vi "FPGA-7842R-Control V2.vi"(0 "Waveform Data":T4, 1 "Current Frame":u16, 2 "Action":T5=enum."Exit", 3 "Laser On Time (Ticks)":u8=13, 5 "Laser Controls":T1 {"STED Power (V)" scale=0.0..10.0}, 7 "Manual Controls":T3={"Galvo 1 Position (I16)"=-280, "Galvo 2 Position (I16)"=-280, "X Axis Voltage (I16)"=0, "Y Axis Voltage (I16)"=0, "Z Axis Voltage (I16)"=0, "Res Mirror Amp (I16)"=0, "Res Mirror Mute"=FALSE, "Upper Shutter"=FALSE, "Lower Shutter"=FALSE}, 9 "Image Acquisition Parameters":T2={"Scan Type"=enum."Sample Scanning", "Scan Mode"=enum."XY", "Fast Axis Frequency (Hz)"=100.0, "Image Format"=128, "Line Accumulations"=1, "Frames Per Capture"=1, "Frames Accumulations"=1, "Image Dimension (um)"=[], "Number of Z Steps"=1, "Z Steps Size (um)"=1.0, "Pixel Size (nm)"=[], "Customized Image Format"=[]} {"Z Steps Size (um)" min=0.0; "Number of Z Steps" min=1; "Frames Accumulations" min=1; "Frames Per Capture" min=1; "Line Accumulations" min=1; "Image Format" items=["64 x 64"=64, "128 x 128"=128, "256 x 256"=256, "512 x 512"=512, "1024 x 1024"=1024, "2048 x 2048"=2048, "Customized..."=0]}, 11 "Initialize":bool, 12 "Unused Axis Offset (I16)":i16, 14 "Laser Delay (Ticks)":u8=6) -> (4 "Shutter Status":cluster{"US Status":bool, "LS Status":bool}, 15 "Initalized":bool)   [LabVIEW 2014]
uses:
  FPGA-7842R-Reference.ctl
  Waveform Data.ctl
  Manual Controls V2.ctl
  Type Defs/Image Acquisition Parameters.ctl
  Laser Controls.ctl
  <vilib>/FPGAPlugInAG/PCIe-7841R/niLvFpga_Open_PCIe-7841R.vi
  <vilib>/Utility/error.llb/Error Cluster From Error Code.vi
  <vilib>/rvi/errors/niLvFpgaAdjustHostInterfaceError.vi
  <vilib>/FPGAPlugInAG/PCIe-7841R/niLvFpga_Run_PCIe-7841R.vi
  <vilib>/FPGAPlugInAG/PCIe-7841R/niLvFpga_Close_PCIe-7841R.vi
  <vilib>/rvi/interface/nirviOpenFPGA/nirviOpenFPGA.xnode
  FPGA Bitfiles/MainSTEDFPGAProj_FPGATarget_WaveformandLaser_sIm2Xng7ncM.lvbitx
  FPGA Target VIs/FPGA-7841R/Waveform and Laser Controls V7.vi
  <vilib>/rvi/interface/nirviReadWriteControl/nirviReadWriteControl.xnode
  FPGA Target VIs/FPGA-7841R/Waveform Scan Parameters.ctl
  <vilib>/rvi/interface/nirviMethod/nirviMethod.xnode
  <vilib>/rvi/interface/nirviCloseFPGA/nirviCloseFPGA.xnode
  NiFpgaLv.dll
panel:
  # "Length"
  # "Height"
  # "XY"
  # "Z"
  # "Length"
  # "Height"
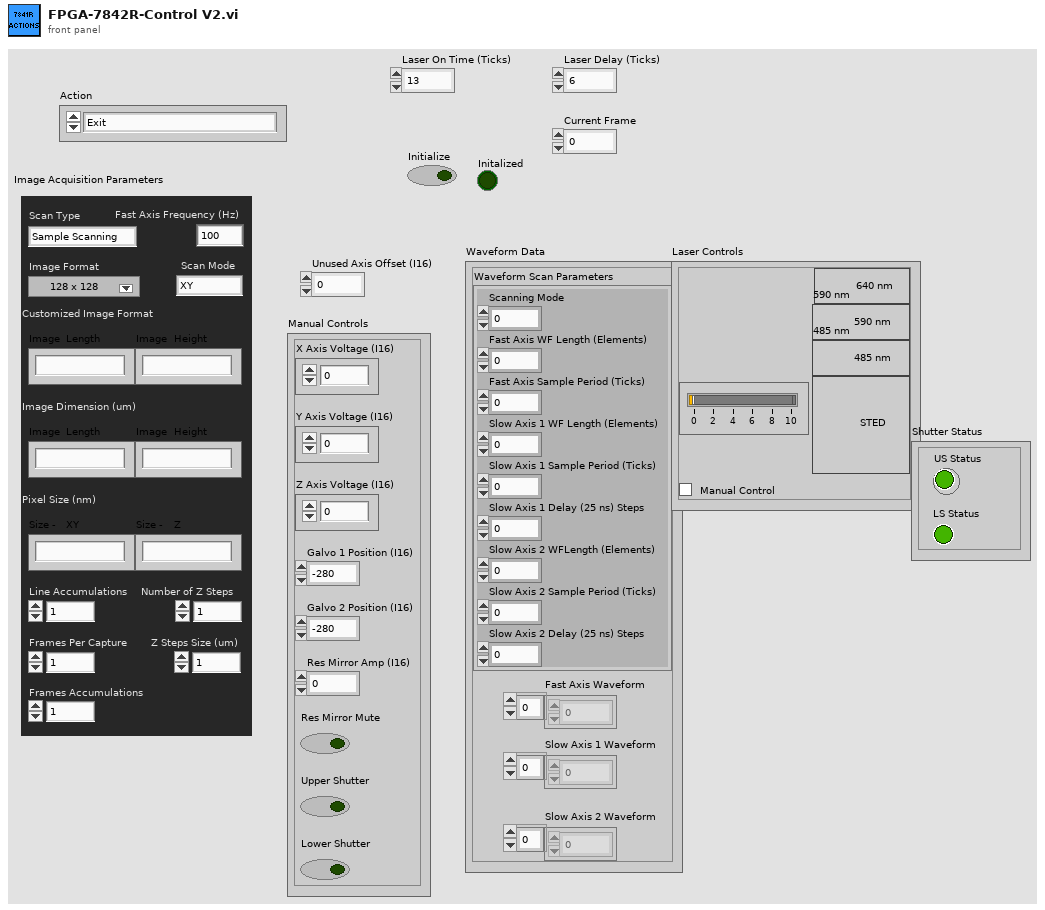
[diagram p1: front panel]
types:
  T1 = typedef "Laser Controls.ctl" = cluster{"STED Power (V)":dbl, "STED":bool, "650 nm":bool, "590 nm":bool, "485 nm":bool, "Manual Control":bool}
  T2 = typedef "Image Acquisition Parameters.ctl" = cluster{"Scan Type":enum16{"Sample Scanning", "Beam Scanning"}, "Scan Mode":enum16{"XY", "XZ", "YZ", "XYZ"}, "Fast Axis Frequency (Hz)":dbl, "Image Format":u16, "Line Accumulations":u16, "Frames Per Capture":u16, "Frames Accumulations":u16, "Image Dimension (um)":dbl[], "Number of Z Steps":u16, "Z Steps Size (um)":dbl, "Pixel Size (nm)":dbl[], "Customized Image Format":dbl[]}
  T3 = typedef "Manual Controls V2.ctl" = cluster{"Galvo 1 Position (I16)":i16, "Galvo 2 Position (I16)":i16, "X Axis Voltage (I16)":i16, "Y Axis Voltage (I16)":i16, "Z Axis Voltage (I16)":i16, "Res Mirror Amp (I16)":i16, "Res Mirror Mute":bool, "Upper Shutter":bool, "Lower Shutter":bool}
  T4 = typedef "Waveform Data.ctl" = cluster{"Waveform Scan Parameters":cluster{"Scanning Mode":u8, "Fast Axis WF Length (Elements)":i32, "Fast Axis Sample Period (Ticks)":u32, "Slow Axis 1 WF Length (Elements)":i32, "Slow Axis 1 Sample Period (Ticks)":u32, "Slow Axis 1 Delay (25 ns) Steps":i32, "Slow Axis 2 WFLength (Elements)":i32, "Slow Axis 2 Sample Period (Ticks)":u32, "Slow Axis 2 Delay (25 ns) Steps":i32}, "Fast Axis Waveform":dbl[], "Slow Axis 1 Waveform":dbl[], "Slow Axis 2 Waveform":dbl[]}
  T5 = typedef "FPGA-7842R-Reference.ctl" = enum16{"Stage Control", "Laser Control", "Unused Axis I16", "Exit", "Set Res Mirror", "Set Galvo", "Current Frame for Capture", "Default", "Close FPGA", "Stop Waveforms", "Start Waveforms", "Shutter Control", "Initialize"}
  T6 = cluster{"Scanning Mode":u8, "Fast Axis WF Length (Elements)":i32, "Fast Axis Sample Period (Ticks)":u32, "Slow Axis 1 WF Length (Elements)":i32, "Slow Axis 1 Sample Period (Ticks)":u32, "Slow Axis 1 Delay (25 ns) Steps":i32, "Slow Axis 2 WFLength (Elements)":i32, "Slow Axis 2 Sample Period (Ticks)":u32, "Slow Axis 2 Delay (25 ns) Steps":i32}
  T7 = cluster{"Res Mirror Amp (I16)":i16, "Res Mirror Mute":bool}
  T8 = typedef "Scan Parameters.ctl" = cluster{"Fast_Ax_Amp_V":dbl, "Fast_Ax_Off_V":dbl, "Slow_Ax_Amp_V":dbl, "Slow_Ax_Off_V ":dbl, "Slow_Ax_Max_V_VperS":dbl, "Slow_Ax1_Del25ns":i32, "Slow_Ax2_Del25ns":i32, "Stage_X_Off_V":dbl, "Stage_Y_Off_V":dbl, "Stage_Z_Off_V":dbl, "Galvo1_Off_V":dbl, "Galvo2_Off_V":dbl, "Last_Scan_Mode":enum16{"XY", "XZ", "YZ", "XYZ"}, "Current_Scan_Mode":enum16{"XY", "XZ", "YZ", "XYZ"}, "Fly_Back_Lines":u16, "Linear_Ramp_End":u32, "Z_Step_I16":i16, "Z_Start_I16":i16, "Laser_States _U32":u32, "590_Voltage_I16":i16, "775_AOM_Volt_I16":i16, "Blanking OFF":bool, "Unused_Axis_I16":i16}
  T9 = cluster{"Upper Shutter Status":bool, "Lower Shutter Status":bool}
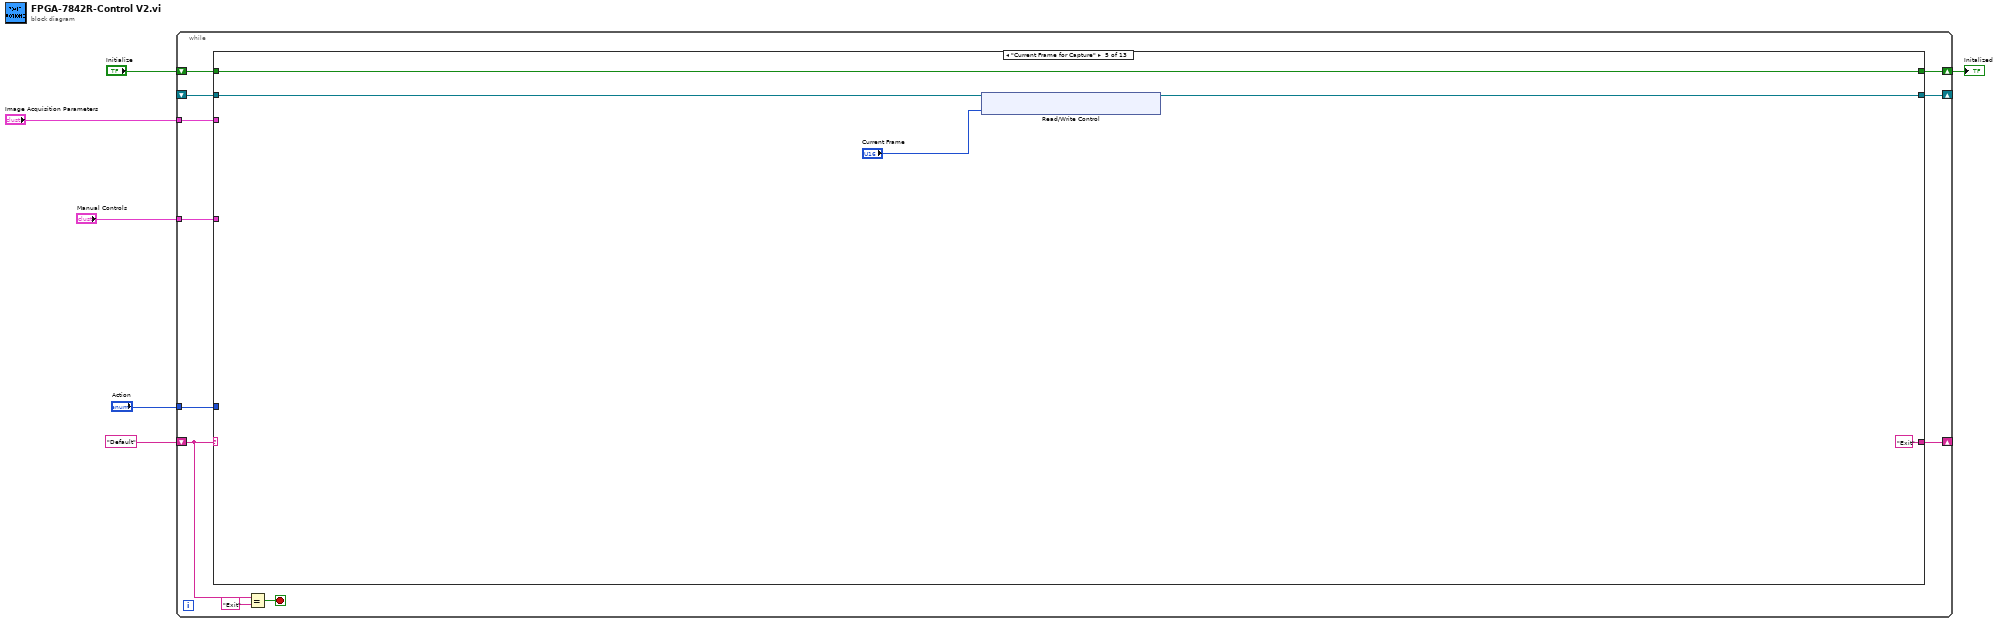
[diagram p0: block diagram]
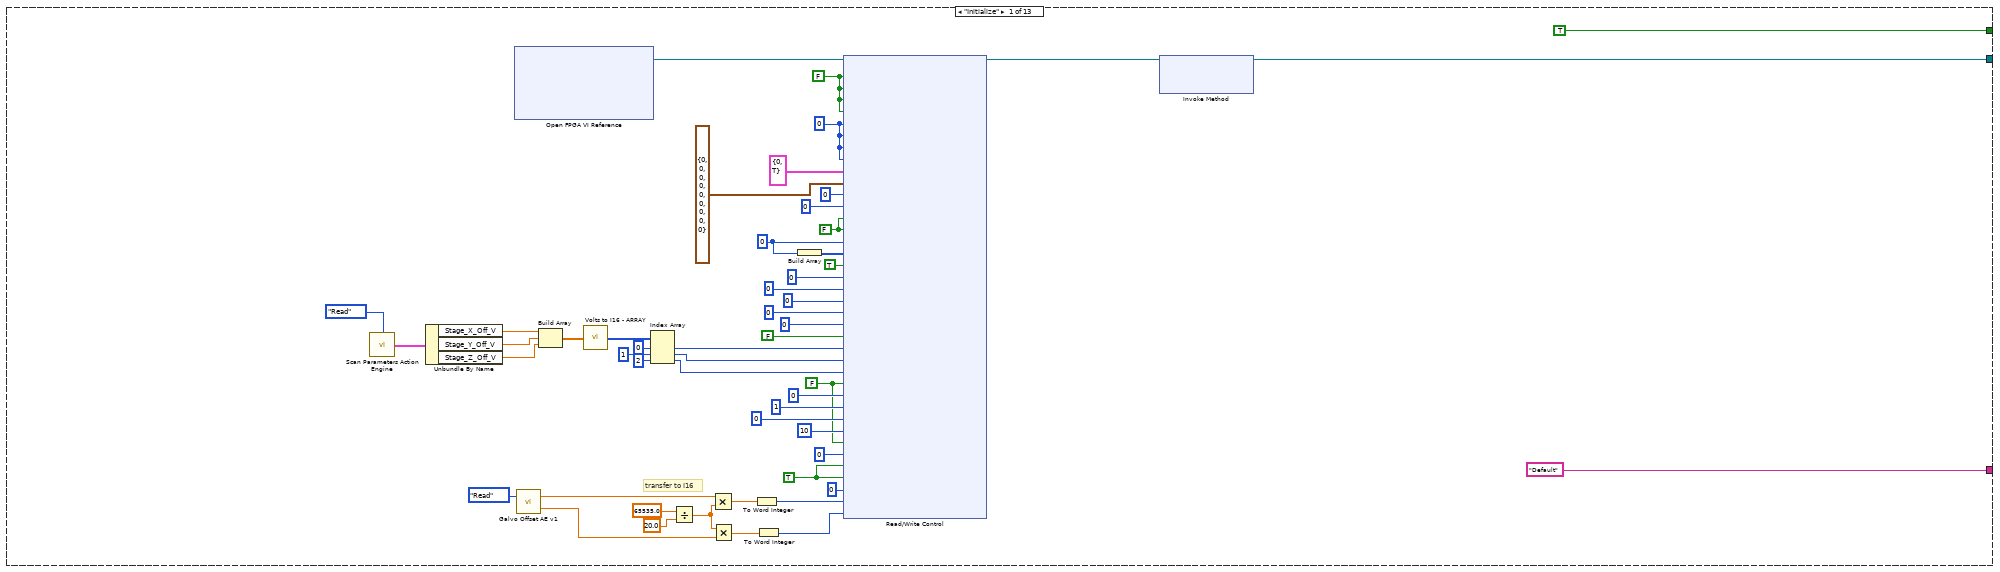
[diagram p2: hidden frame]
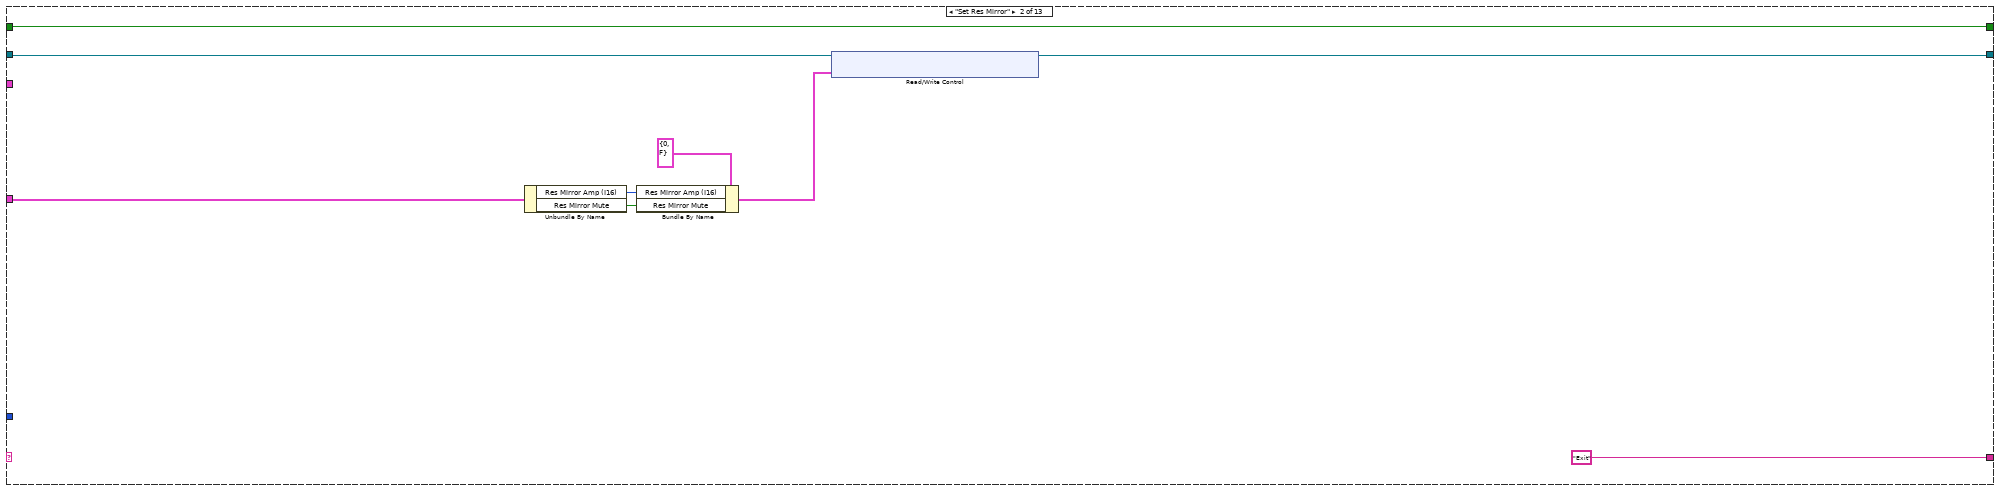
[diagram p3: hidden frame]
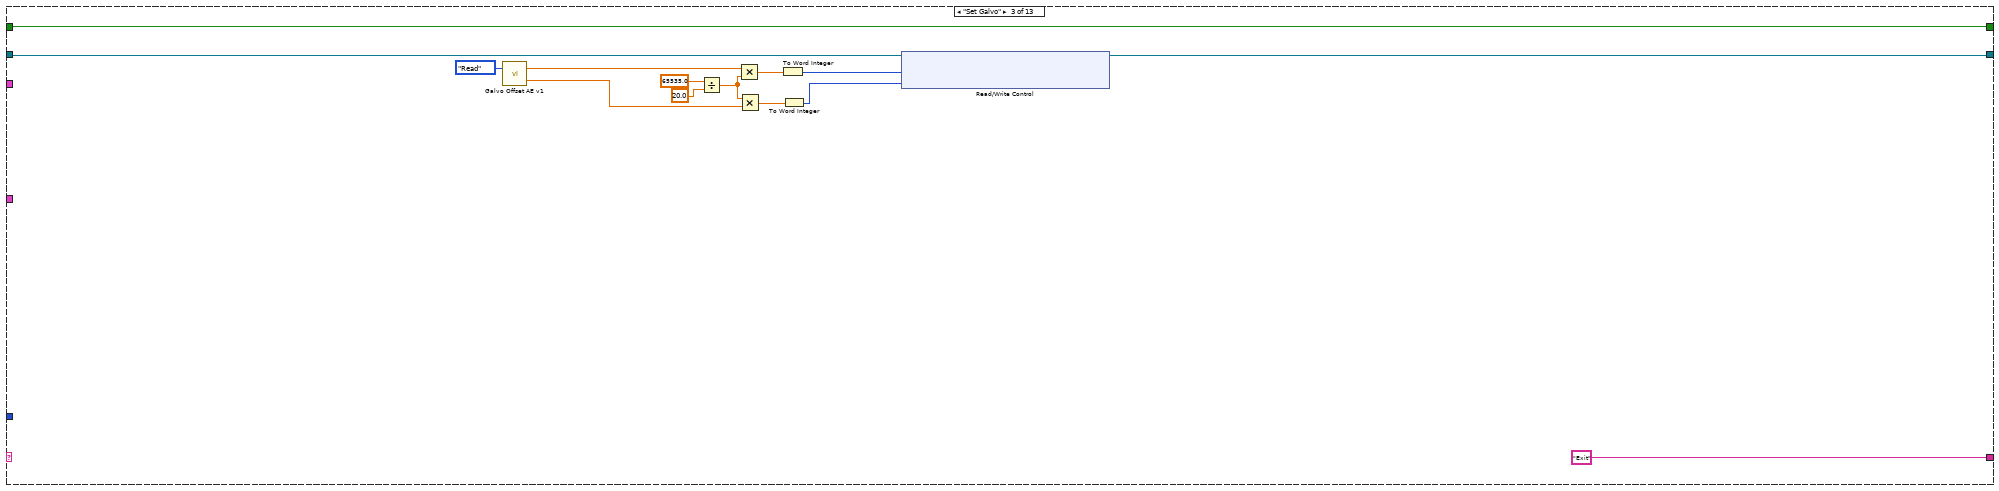
[diagram p4: hidden frame]
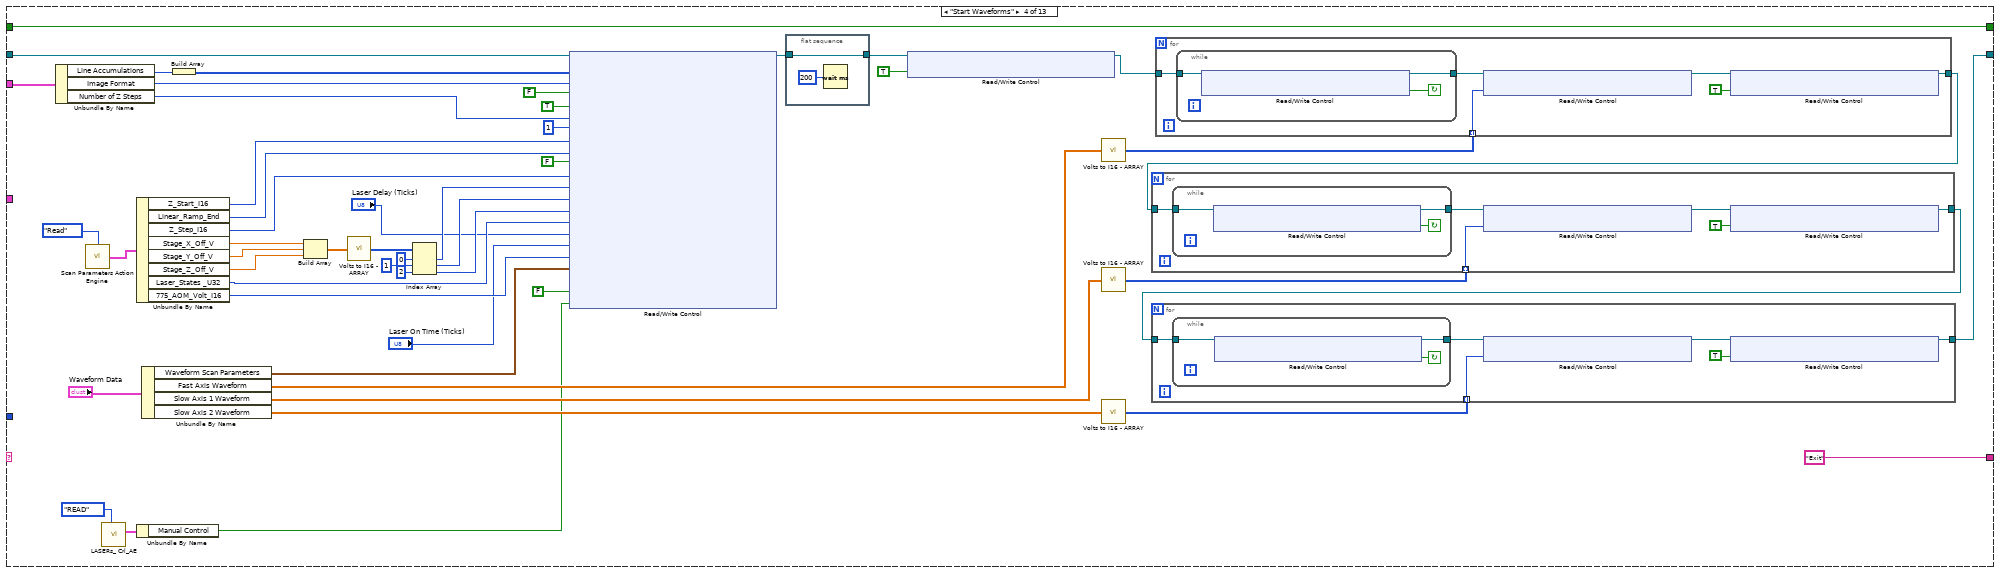
[diagram p5: hidden frame]
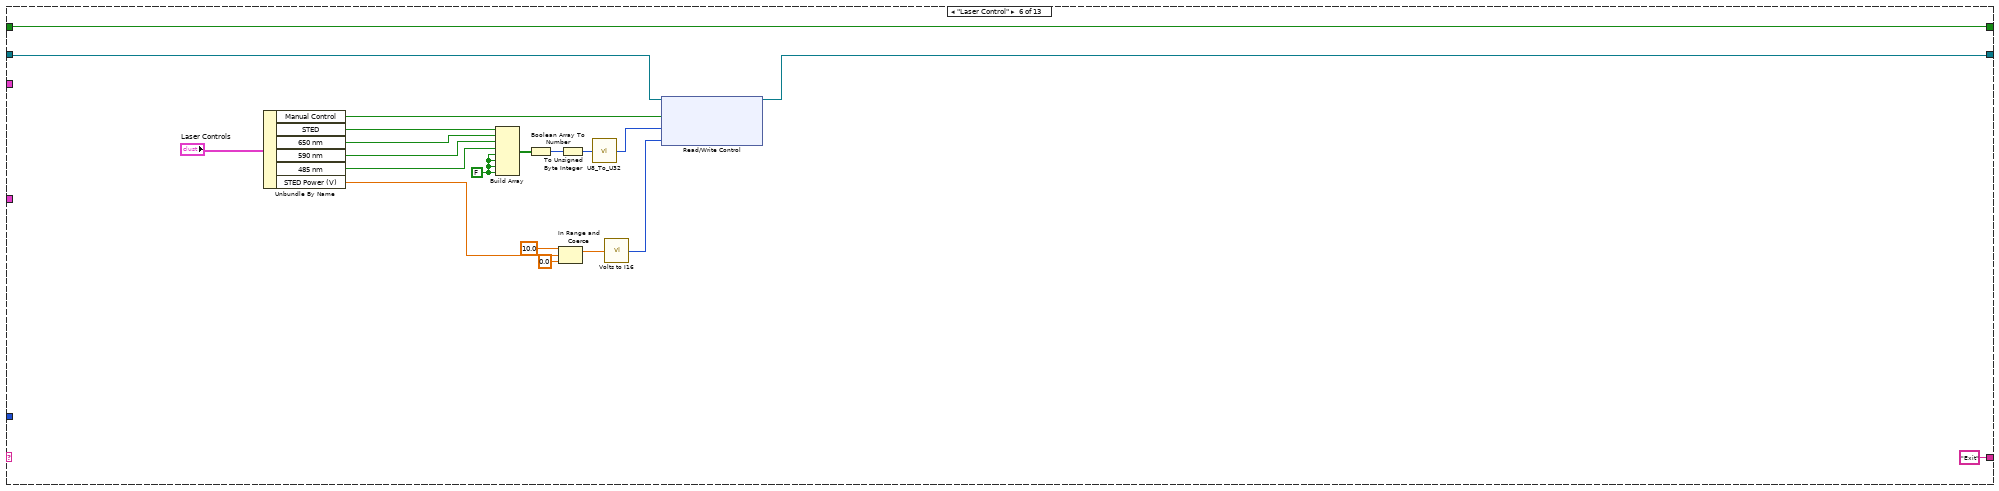
[diagram p6: hidden frame]
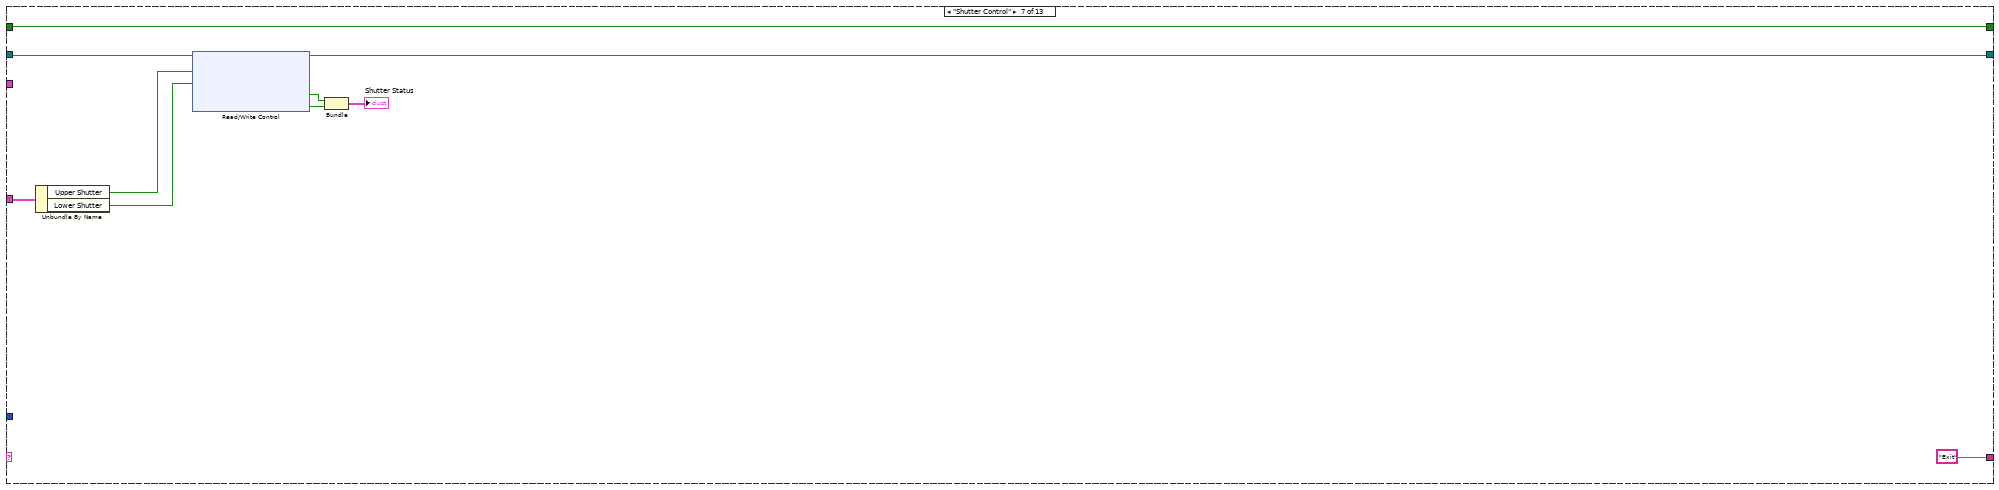
[diagram p7: hidden frame]
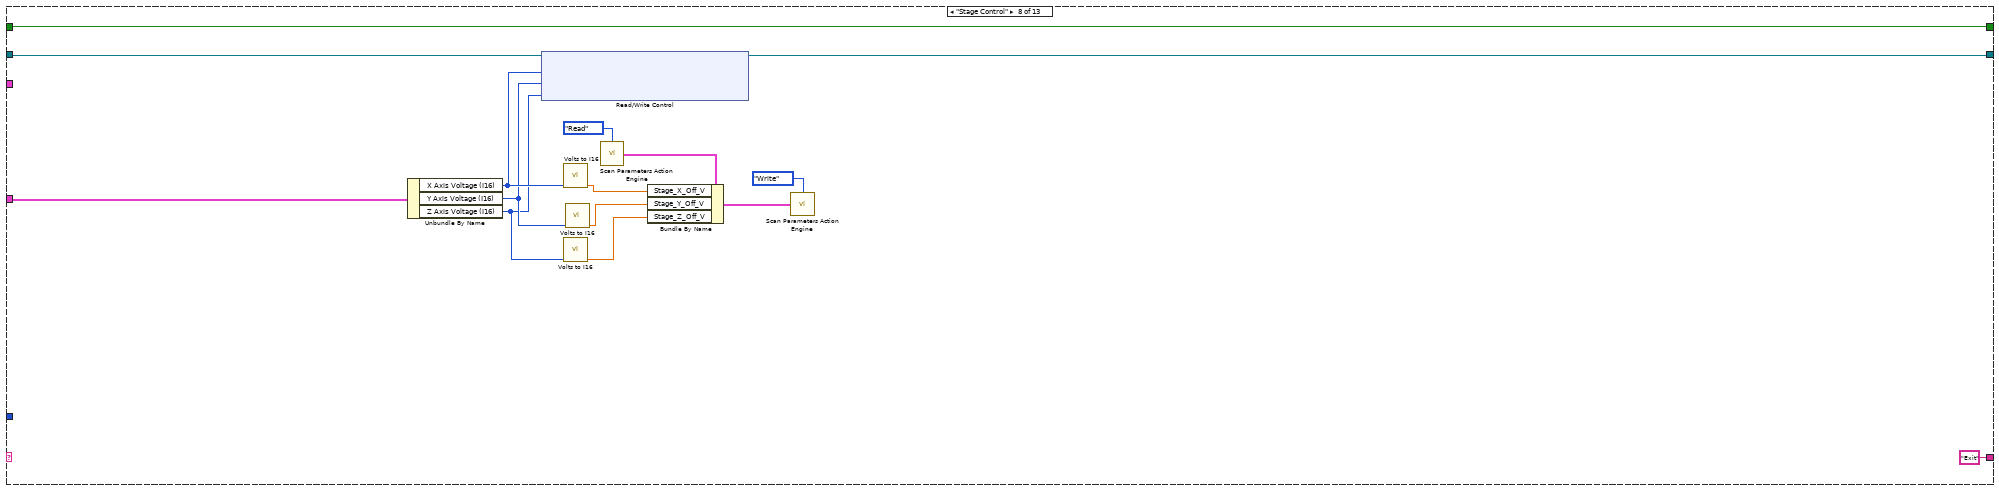
[diagram p8: hidden frame]
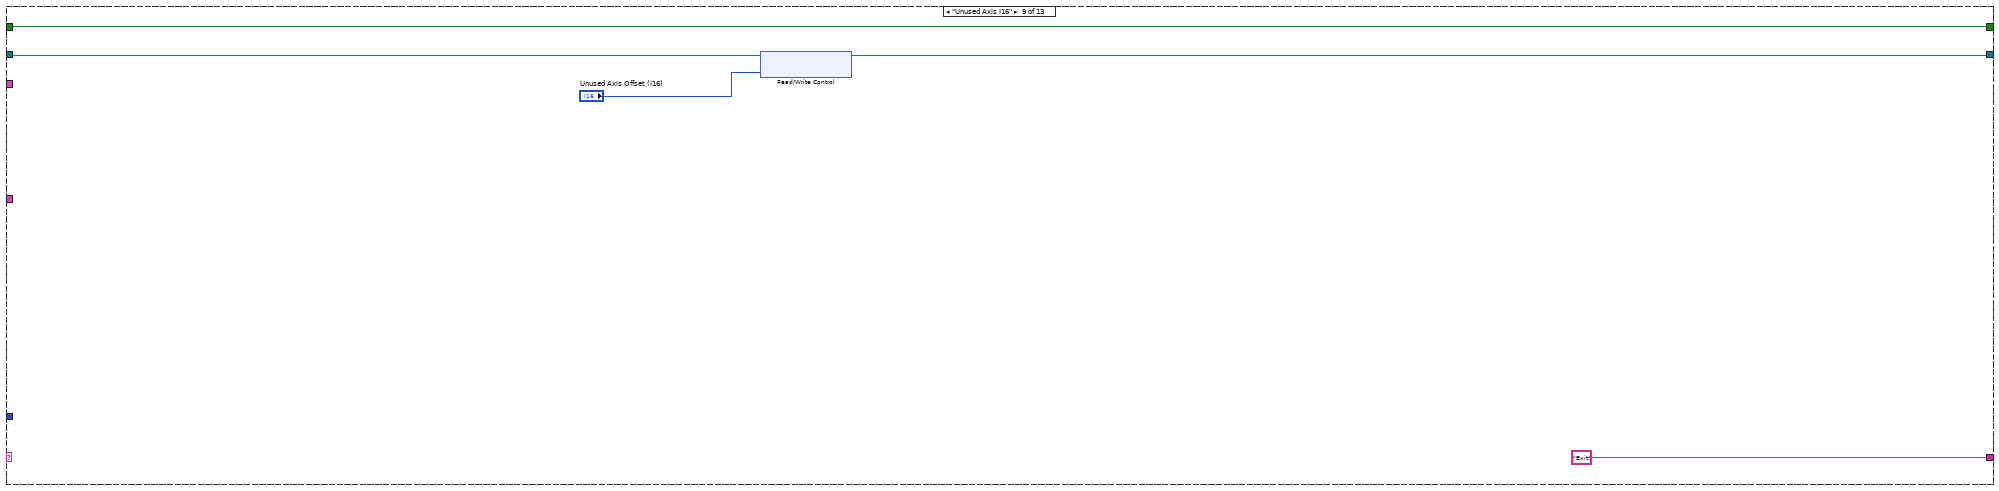
[diagram p9: hidden frame]
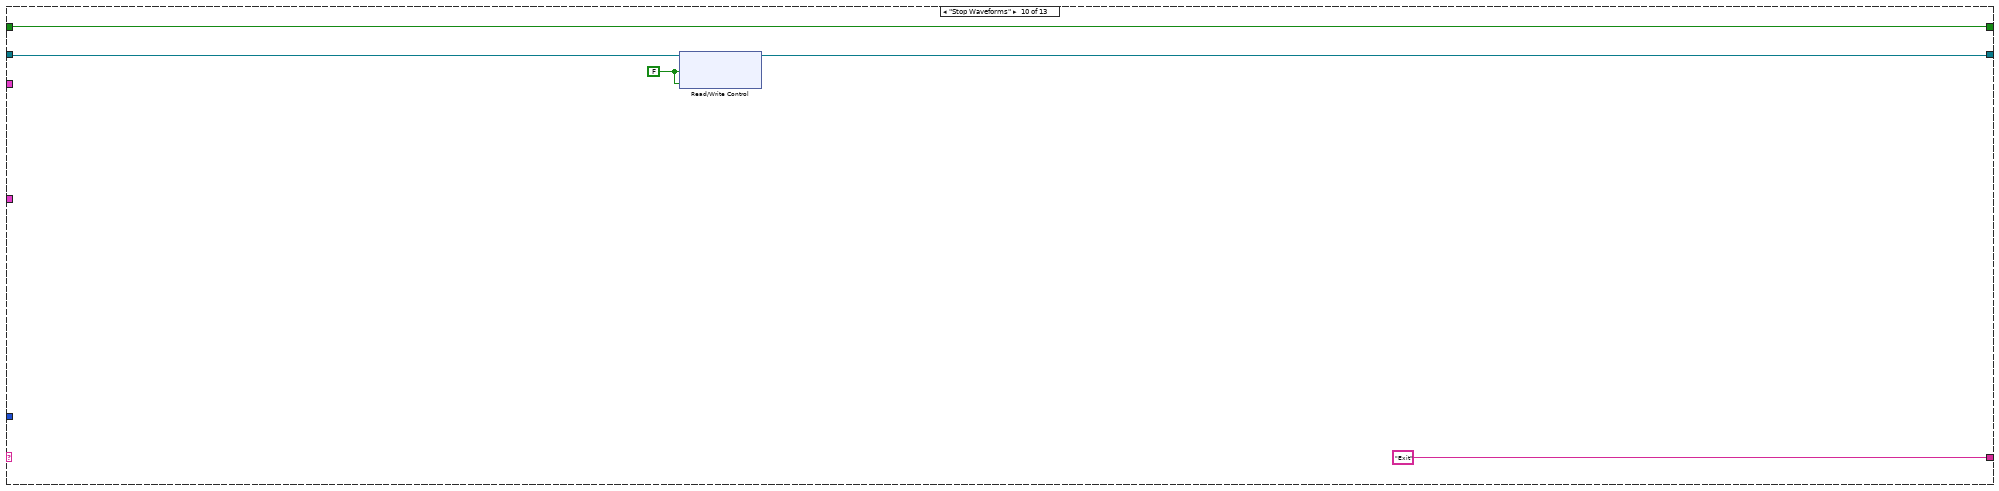
[diagram p10: hidden frame]
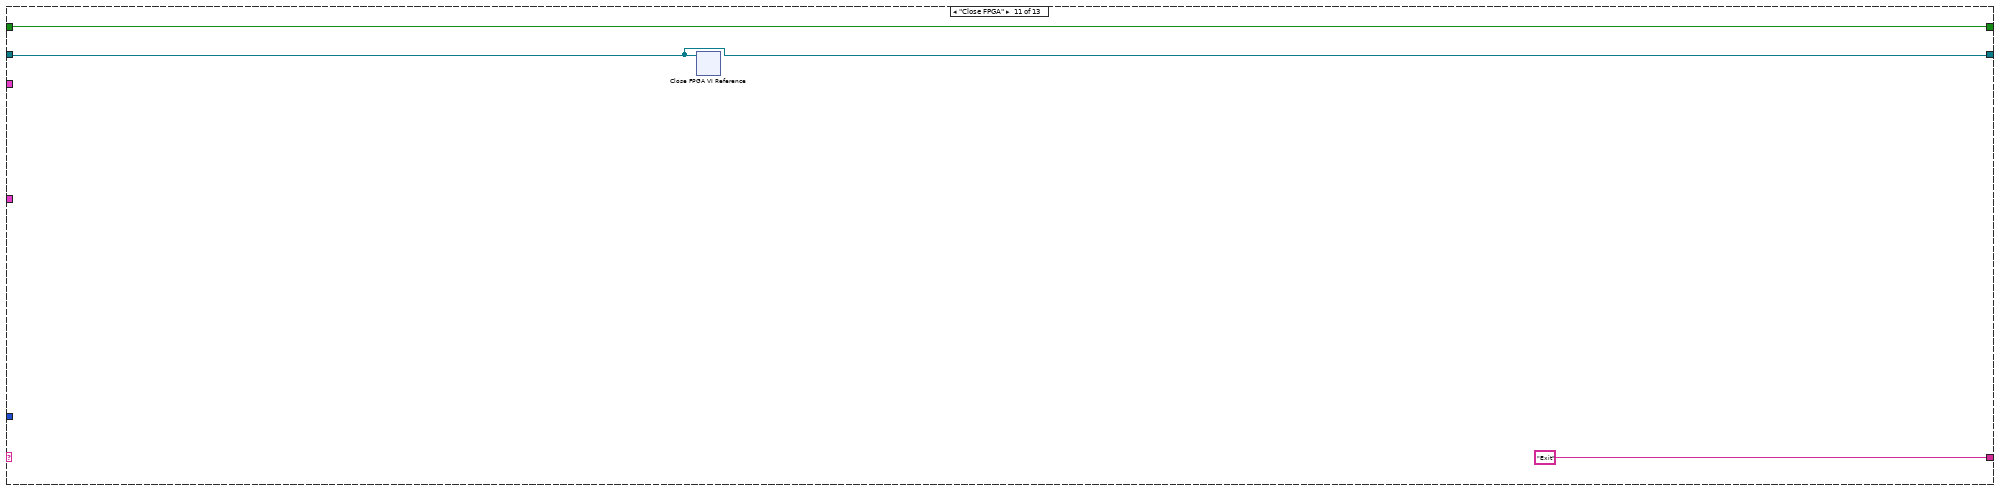
[diagram p11: hidden frame]
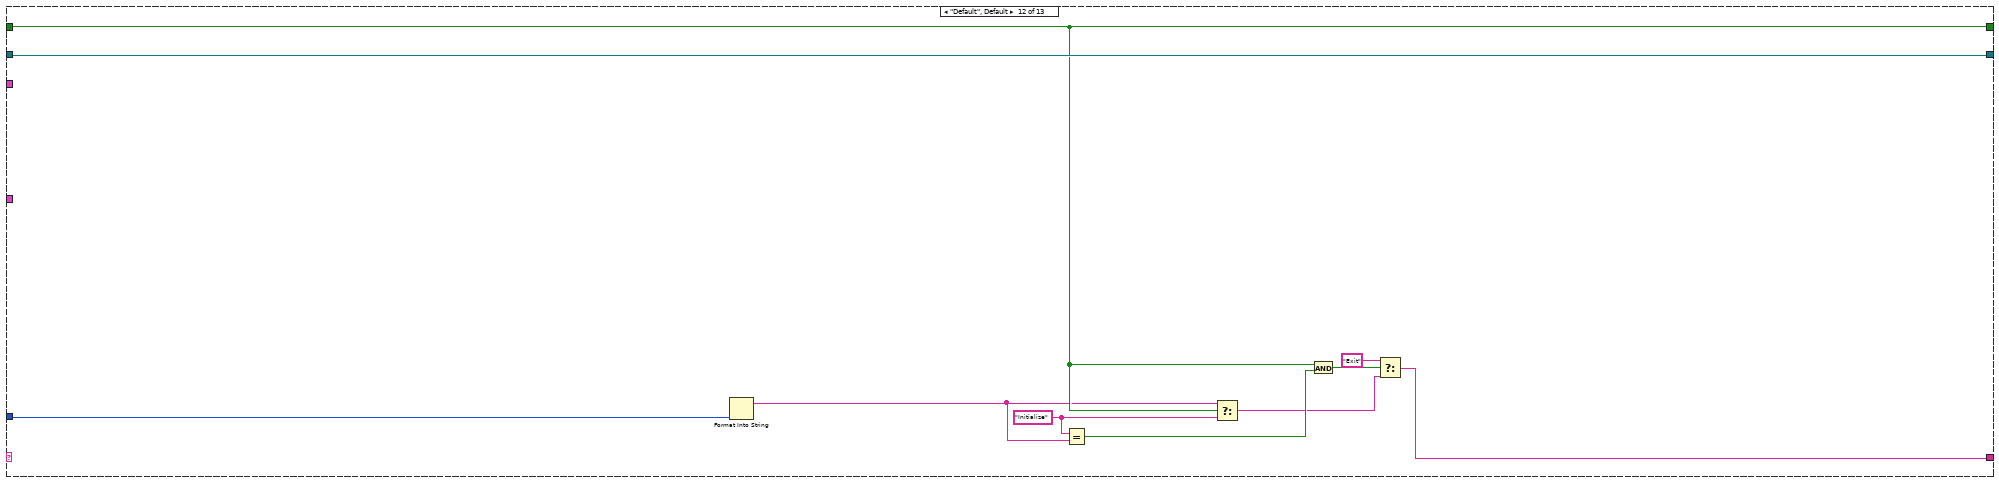
[diagram p12: hidden frame]
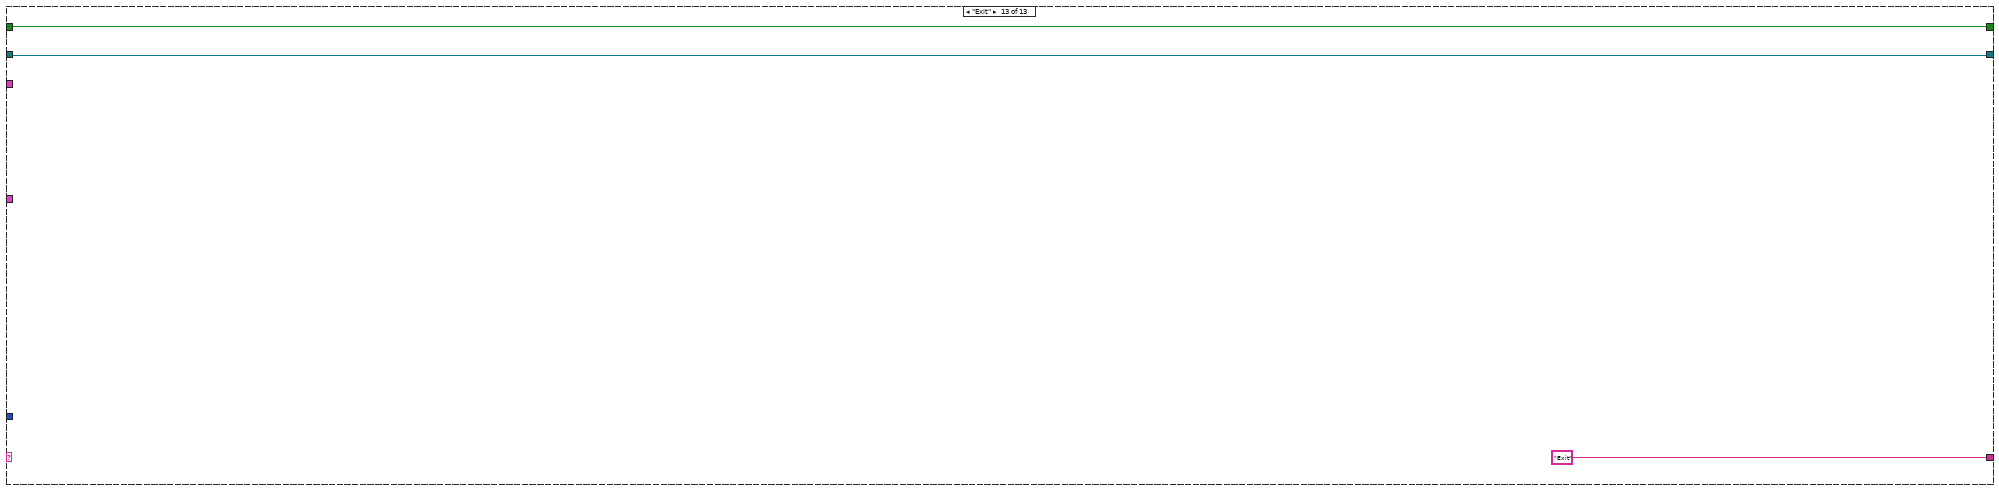
[diagram p13: hidden frame]
diagram:
  n1 = while {
    shift-right: [w17] -> _
    shift-left: _ -> [w16]
    shift-right: [w14] -> _
    shift-left: "Default" -> [w13]
    tunnel: "Action" -> [w15]
    shift-right: [w10] -> w3
    shift-left: "Initialize" -> [w9]
    tunnel: "Manual Controls" -> [w8]
    tunnel: "Image Acquisition Parameters" -> [w7]
    stop <- w11 stop-if-true
    n2 = case shown="\"Current Frame for Capture\"" w13 {
      tunnel: [w60 w75 w89 w132 w175 w193 w205 w218 w224 w231 w233 w245 w247] -> w17
      tunnel: w16 -> [_ w76 w90 w135 w176 w194 w206 w219 w225 w232 w233 w245 w247]
      tunnel: w15 -> [_ _ _ _ _ _ _ _ _ _ _ w244 _]
      tunnel: ["Default" ("f") "Exit" ("f") "Exit" ("f") "Exit" ("f") "Exit" ("f") "Exit" ("f") "Exit" ("f") "Exit" ("f") "Exit" ("f") "Exit" ("f") "Exit" ("f") w238 "Exit" ("f")] -> w14
      tunnel: [TRUE w78 w92 w137 w177 w196 w207 w221 w227 w230 w235 w243 w248] -> w10
      tunnel: w9 -> [_ w78 w92 w137 w177 w196 w207 w221 w227 w230 w235 w243 w248]
      tunnel: w8 -> [_ w74 _ _ _ _ w200 w220 _ _ _ _ _]
      tunnel: w7 -> [_ _ _ w126 _ _ _ _ _ _ _ _ _]
      frame "Initialize" {
        w29 = TRUE ("Upper Shutter Command")
        w31 = FALSE ("Blanking Off/Manual")
        w56 = u16 0 ("Number of Lines")
        w58 = FALSE ("Reset Position Error")
        w69 = i16 0 ("Fast Axis Waveform Element")
        w68 = FALSE ("WF 1 Data Loaded")
        # "transfer to I16"
        n3 = call "Scan Parameters Action Engine.vi"("Action"=enum16{"Read", "Write"}."Read") -> ("Scan Parameters OUT"=w47:T8)  [unwired: 14 in]
        n4 = Unbundle By Name(w47) -> ("Stage_X_Off_V"=w46:dbl, "Stage_Y_Off_V"=w44:dbl, "Stage_Z_Off_V"=w45:dbl)
        n5 = xnode "Open FPGA VI Reference"() -> ("FPGA VI Reference Out"=w59:refnum<k20>)  [unwired: 2 in, 1 out]
        n6 = call "Galvo Offset AE v1.vi"("Action"=enum16{"Read", "Write"}."Read") -> ("Galvo 2 Offset Out"=w18:dbl, "Galvo 1 Offset Out"=w19:dbl)  [unwired: 1 in]
        n7 = Build Array(w46, w44, w45) -> (w43:dbl[])
        n8 = call "Volts to I16 - ARRAY.vi"("Voltage (V)"=w43) -> ("I16"=w42:i16[])  [unwired: 14 in]
        n9 = Index Array(array=w42, index #1=0 ("index"), index #2=1 ("index"), index #3=2 ("index")) -> (element #1=w38:i16, element #2=w36:i16, element #3=w37:i16)
        n10 = Divide(x=65535.0, y=20.0 ("x")) -> (x/y=w23:dbl)
        n11 = Multiply(x=w19, y=w23) -> (x*y=w25:dbl)
        n12 = Multiply(x=w23, y=w18) -> (x*y=w22:dbl)
        n13 = To Word Integer(number=w25) -> (16bit integer=w24:i16)
        n14 = To Word Integer(number=w22) -> (16bit integer=w21:i16)
        n15 = Build Array(w56) -> (w55:u16[])
        n16 = xnode "Read/Write Control"("FPGA VI Reference In"=w59, "WF 1 Data Loaded"=w68, "WF 2 Data Loaded"=w68, "WF 3 Data Loaded"=w68, "Start Waveforms"=w68, "Fast Axis Waveform Element"=w69, "Slow Axis 1 Waveform Element"=w69, "Slow Axis 2 Waveform Element"=w69, "Unused Axis Offset"=w69, "Resonant Mirror"=T7 {"Res Mirror Amp (I16)"=0, "Res Mirror Mute"=TRUE} ("Resoance Mirror"), "Waveform Scan Parameters"=T6 {"Scanning Mode"=0, "Fast Axis WF Length (Elements)"=0, "Fast Axis Sample Period (Ticks)"=0, "Slow Axis 1 WF Length (Elements)"=0, "Slow Axis 1 Sample Period (Ticks)"=0, "Slow Axis 1 Delay (25 ns) Steps"=0, "Slow Axis 2 WFLength (Elements)"=0, "Slow Axis 2 Sample Period (Ticks)"=0, "Slow Axis 2 Delay (25 ns) Steps"=0}, "Galvo 2 Position (I16)"=i16 0, "Galvo 1 Position (I16)"=i16 0, "Reset Position Error"=w58, "Frame Trigger"=w58, "Number of Lines"=w56, "Accums Per Line"=w55, "Stop Sync Signal"=TRUE, "Z Step Size (I16)"=i16 0, "Number of Z Steps"=u8 0, "Frames Per Z Step"=u8 0, "Z Stack Start Position (I16)"=i16 0, "End of Linear Ramp"=u32 0, "End Linear Ramp"=FALSE, "X Piezo Axis"=w38, "Y Piezo Axis"=w36, "Z Piezo Axis"=w37, "Blanking Off/Manual"=w31, "Laser States"=u32 0, "Laser Delay (Ticks)"=u8 1, "Sequences"=u8 0, "Laser On Time (Ticks)"=u8 10, "Laser Blank Trigger"=w31, "775 AOM (I16)"=i16 0 ("590 Analog Voltage (I16)"), "Upper Shutter Command"=w29, "Lower Shutter Command"=w29, "Current Frame"=u8 0, "Galvo 1 Position (I16)"=w24, "Galvo 2 Position (I16)"=w21) -> ("FPGA VI Reference Out"=w65:refnum<k20>)  [unwired: 1 in, 1 out]
        n17 = xnode "Invoke Method"("FPGA VI Reference In"=w65) -> ("FPGA VI Reference Out"=w60:refnum<k20>)  [unwired: 2 in, 1 out]
      }
      frame "Set Res Mirror" {
        n18 = Unbundle By Name(w74) -> ("Res Mirror Amp (I16)"=w73:i16, "Res Mirror Mute"=w72:bool)
        n19 = Bundle By Name(cluster=T7 {"Res Mirror Amp (I16)"=0, "Res Mirror Mute"=FALSE} ("Resoance Mirror"), "Res Mirror Amp (I16)"=w73, "Res Mirror Mute"=w72) -> (w70:T7)
        n20 = xnode "Read/Write Control"("FPGA VI Reference In"=w76, "Resonant Mirror"=w70) -> ("FPGA VI Reference Out"=w75:refnum<k20>)  [unwired: 1 in, 1 out]
      }
      frame "Set Galvo" {
        n21 = call "Galvo Offset AE v1.vi"("Action"=enum16{"Read", "Write"}."Read") -> ("Galvo 2 Offset Out"=w79:dbl, "Galvo 1 Offset Out"=w80:dbl)  [unwired: 1 in]
        n22 = Divide(x=65535.0, y=20.0 ("x")) -> (x/y=w84:dbl)
        n23 = Multiply(x=w80, y=w84) -> (x*y=w85:dbl)
        n24 = Multiply(x=w84, y=w79) -> (x*y=w83:dbl)
        n25 = To Word Integer(number=w85) -> (16bit integer=w81:i16)
        n26 = To Word Integer(number=w83) -> (16bit integer=w82:i16)
        n27 = xnode "Read/Write Control"("FPGA VI Reference In"=w90, "Galvo 1 Position (I16)"=w81, "Galvo 2 Position (I16)"=w82) -> ("FPGA VI Reference Out"=w89:refnum<k20>)  [unwired: 1 in, 1 out]
      }
      frame "Start Waveforms" {
        n28 = Unbundle By Name(w126) -> ("Line Accumulations"=w124:u16, "Image Format"=w125:u16, "Number of Z Steps"=w115:u16)
        n29 = call "Scan Parameters Action Engine.vi"("Action"=enum16{"Read", "Write"}."Read") -> ("Scan Parameters OUT"=w119:T8)  [unwired: 14 in]
        n30 = call "LASERs_ Crl_AE.vi"("Action"=enum16{"READ", "WRITE"}."READ") -> ("Laser Parameters Out"=w94:T1)  [unwired: 10 in]
        n31 = Unbundle By Name(w119) -> ("Z_Start_I16"=w117:i16, "Linear_Ramp_End"=w118:u32, "Z_Step_I16"=w114:i16, "Stage_X_Off_V"=w107:dbl, "Stage_Y_Off_V"=w106:dbl, "Stage_Z_Off_V"=w105:dbl, "Laser_States _U32"=w101:u32, "775_AOM_Volt_I16"=w100:i16)
        n32 = Unbundle By Name(w94) -> ("Manual Control"=w93:bool)
        n33 = Unbundle By Name("Waveform Data") -> ("Waveform Scan Parameters"=w99:T6, "Fast Axis Waveform"=w139:dbl[], "Slow Axis 1 Waveform"=w131:dbl[], "Slow Axis 2 Waveform"=w138:dbl[])
        n34 = Build Array(w124) -> (w123:u16[])
        n35 = Build Array(w107, w106, w105) -> (w112:dbl[])
        n36 = call "Volts to I16 - ARRAY.vi"("Voltage (V)"=w112) -> ("I16"=w111:i16[])  [unwired: 14 in]
        n37 = Index Array(array=w111, index #1=0 ("index"), index #2=1 ("index"), index #3=2 ("index")) -> (element #1=w104:i16, element #2=w103:i16, element #3=w102:i16)
        n38 = xnode "Read/Write Control"("FPGA VI Reference In"=w135, "Accums Per Line"=w123, "Number of Lines"=w125, "Frame Trigger"=FALSE, "Stop Sync Signal"=TRUE, "Number of Z Steps"=w115, "Frames Per Z Step"=u16 1, "Z Stack Start Position (I16)"=w117, "End of Linear Ramp"=w118, "End Linear Ramp"=FALSE, "Z Step Size (I16)"=w114, "X Piezo Axis"=w104, "Y Piezo Axis"=w103, "Z Piezo Axis"=w102, "Laser States"=w101, "Laser Delay (Ticks)"="Laser Delay (Ticks)", "Laser On Time (Ticks)"="Laser On Time (Ticks)", "775 AOM (I16)"=w100, "Waveform Scan Parameters"=w99, "Frame Trigger"=FALSE, "Blanking Off/Manual"=w93) -> ("FPGA VI Reference Out"=w133:refnum<k20>)  [unwired: 1 in, 2 out]
        n39 = flat-sequence {
          tunnel: [w145] -> w134
          tunnel: w133 -> [w145]
          frame #0 {
            n40 = Wait (ms)(milliseconds to wait=u32 200) -> ()  [unwired: 1 out]
          }
        }
        n41 = xnode "Read/Write Control"("FPGA VI Reference In"=w134, "Start Waveforms"=TRUE) -> ("FPGA VI Reference Out"=w140:refnum<k20>)  [unwired: 1 in, 1 out]
        n42 = call "Volts to I16 - ARRAY.vi"("Voltage (V)"=w139) -> ("I16"=w143:i16[])  [unwired: 14 in]
        n43 = call "Volts to I16 - ARRAY.vi"("Voltage (V)"=w131) -> ("I16"=w129:i16[])  [unwired: 14 in]
        n44 = call "Volts to I16 - ARRAY.vi"("Voltage (V)"=w138) -> ("I16"=w130:i16[])  [unwired: 14 in]
        n45 = for {
          tunnel: w140 -> [w168]
          tunnel: [w166] -> w142
          tunnel: w143 -> [w164] mode=indexing
          n46 = while {
            tunnel: w168 -> [w172]
            tunnel: [w171] -> w167
            stop <- w170 continue-if-true
            n47 = xnode "Read/Write Control"("FPGA VI Reference In"=w172) -> ("FPGA VI Reference Out"=w171:refnum<k20>, "WF 1 Data Loaded"=w170:bool)  [unwired: 1 in, 1 out]
          }
          n48 = xnode "Read/Write Control"("FPGA VI Reference In"=w167, "Fast Axis Waveform Element"=w164) -> ("FPGA VI Reference Out"=w169:refnum<k20>)  [unwired: 1 in, 1 out]
          n49 = xnode "Read/Write Control"("FPGA VI Reference In"=w169, "WF 1 Data Loaded"=TRUE ("Host Data Loaded")) -> ("FPGA VI Reference Out"=w166:refnum<k20>)  [unwired: 1 in, 1 out]
        }
        n50 = for {
          tunnel: w142 -> [w159]
          tunnel: [w157] -> w113
          tunnel: w129 -> [w155] mode=indexing
          n51 = while {
            tunnel: w159 -> [w163]
            tunnel: [w162] -> w158
            stop <- w161 continue-if-true
            n52 = xnode "Read/Write Control"("FPGA VI Reference In"=w163) -> ("FPGA VI Reference Out"=w162:refnum<k20>, "WF 2 Data Loaded"=w161:bool)  [unwired: 1 in, 1 out]
          }
          n53 = xnode "Read/Write Control"("FPGA VI Reference In"=w158, "Slow Axis 1 Waveform Element"=w155) -> ("FPGA VI Reference Out"=w160:refnum<k20>)  [unwired: 1 in, 1 out]
          n54 = xnode "Read/Write Control"("FPGA VI Reference In"=w160, "WF 2 Data Loaded"=TRUE ("Host Data Loaded")) -> ("FPGA VI Reference Out"=w157:refnum<k20>)  [unwired: 1 in, 1 out]
        }
        n55 = for {
          tunnel: w113 -> [w150]
          tunnel: [w148] -> w132
          tunnel: w130 -> [w146] mode=indexing
          n56 = while {
            tunnel: w150 -> [w154]
            tunnel: [w153] -> w149
            stop <- w152 continue-if-true
            n57 = xnode "Read/Write Control"("FPGA VI Reference In"=w154) -> ("FPGA VI Reference Out"=w153:refnum<k20>, "WF 3 Data Loaded"=w152:bool)  [unwired: 1 in, 1 out]
          }
          n58 = xnode "Read/Write Control"("FPGA VI Reference In"=w149, "Slow Axis 2 Waveform Element"=w146) -> ("FPGA VI Reference Out"=w151:refnum<k20>)  [unwired: 1 in, 1 out]
          n59 = xnode "Read/Write Control"("FPGA VI Reference In"=w151, "WF 3 Data Loaded"=TRUE ("Host Data Loaded")) -> ("FPGA VI Reference Out"=w148:refnum<k20>)  [unwired: 1 in, 1 out]
        }
      }
      frame "Current Frame for Capture" {
        n60 = xnode "Read/Write Control"("FPGA VI Reference In"=w176, "Current Frame"="Current Frame") -> ("FPGA VI Reference Out"=w175:refnum<k20>)  [unwired: 1 in, 1 out]
      }
      frame "Laser Control" {
        w187 = FALSE ("element")
        n61 = Unbundle By Name("Laser Controls") -> ("Manual Control"=w195:bool, "STED"=w184:bool, "650 nm"=w183:bool, "590 nm"=w182:bool, "485 nm"=w181:bool, "STED Power (V)"=w180:dbl)
        n62 = Build Array(w184, w183, w182, w181, w187, w187, w187, w187) -> (w185:bool[])
        n63 = Boolean Array To Number(Boolean array=w185) -> (number=w186:u32)
        n64 = In Range and Coerce(upper limit=10.0, x=w180, lower limit=0.0) -> (coerced(x)=w191:dbl)  [unwired: 1 out]
        n65 = To Unsigned Byte Integer(number=w186) -> (unsigned 8bit integer=w188:u8)
        n66 = call "U8_To_U32.vi"("U8 IN"=w188) -> ("U32 OUT"=w179:u32)  [unwired: 13 in, 1 out]
        n67 = call "Volts to I16.vi"("Voltage (V)"=w191) -> ("I16"=w178:i16)  [unwired: 13 in, 1 out]
        n68 = xnode "Read/Write Control"("FPGA VI Reference In"=w194, "Blanking Off/Manual"=w195, "Laser States"=w179, "775 AOM (I16)"=w178) -> ("FPGA VI Reference Out"=w193:refnum<k20>)  [unwired: 1 in, 1 out]
      }
      frame "Shutter Control" {
        n69 = Unbundle By Name(w200) -> ("Upper Shutter"=w198:bool, "Lower Shutter"=w199:bool)
        n70 = xnode "Read/Write Control"("FPGA VI Reference In"=w206, "Upper Shutter Command"=w198, "Lower Shutter Command"=w199) -> ("FPGA VI Reference Out"=w205:refnum<k20>, "Upper Shutter Status"=w203:bool, "Lower Shutter Status"=w202:bool)  [unwired: 1 in, 1 out]
        n71 = Bundle("Upper Shutter Status"=w203, "Lower Shutter Status"=w202) -> (→"Shutter Status":T9)  [unwired: 1 in]
      }
      frame "Stage Control" {
        n72 = Unbundle By Name(w220) -> ("X Axis Voltage (I16)"=w215:i16, "Y Axis Voltage (I16)"=w211:i16, "Z Axis Voltage (I16)"=w210:i16)
        n73 = xnode "Read/Write Control"("FPGA VI Reference In"=w219, "X Piezo Axis"=w215, "Y Piezo Axis"=w211, "Z Piezo Axis"=w210) -> ("FPGA VI Reference Out"=w218:refnum<k20>)  [unwired: 1 in, 1 out]
        n74 = call "Volts to I16.vi"("Volatge (I16)"=w215) -> ("Voltage (V)"=w214:dbl)  [unwired: 13 in, 1 out]
        n75 = call "Volts to I16.vi"("Volatge (I16)"=w210) -> ("Voltage (V)"=w212:dbl)  [unwired: 13 in, 1 out]
        n76 = call "Volts to I16.vi"("Volatge (I16)"=w211) -> ("Voltage (V)"=w213:dbl)  [unwired: 13 in, 1 out]
        n77 = call "Scan Parameters Action Engine.vi"("Action"=enum16{"Read", "Write"}."Read") -> ("Scan Parameters OUT"=w216:T8)  [unwired: 14 in]
        n78 = Bundle By Name(cluster=w216, "Stage_X_Off_V"=w214, "Stage_Y_Off_V"=w213, "Stage_Z_Off_V"=w212) -> (w208:T8)
        n79 = call "Scan Parameters Action Engine.vi"("Action"=enum16{"Read", "Write"}."Write", "Scan Parameters IN"=w208) -> ()  [unwired: 13 in, 1 out]
      }
      frame "Unused Axis I16" {
        n80 = xnode "Read/Write Control"("FPGA VI Reference In"=w225, "Unused Axis Offset"="Unused Axis Offset (I16)") -> ("FPGA VI Reference Out"=w224:refnum<k20>)  [unwired: 1 in, 1 out]
      }
      frame "Stop Waveforms" {
        w228 = FALSE ("Start Waveforms")
        n81 = xnode "Read/Write Control"("FPGA VI Reference In"=w232, "Start Waveforms"=w228, "Stop Sync Signal"=w228) -> ("FPGA VI Reference Out"=w231:refnum<k20>)  [unwired: 1 in, 1 out]
      }
      frame "Close FPGA" {
        n82 = xnode "Close FPGA VI Reference"("FPGA VI Reference In"=w233) -> ()  [unwired: 1 in, 1 out]
      }
      frame "Default", Default {
        w237 = "Initialize" ("f")
        n83 = Format Into String(w244) -> (resulting string=w236:string)  [unwired: 3 in, 1 out]
        n84 = Equal?(x=w237, y=w236) -> (x = y?=w242:bool)
        n85 = Select(t=w236, s=w243, f=w237) -> (s? t:f=w239:string)
        n86 = And(x=w243, y=w242) -> (x .and. y?=w241:bool)
        n87 = Select(t="Exit" ("y"), s=w241, f=w239) -> (s? t:f=w238:string)
      }
      frame "Exit" {
      }
    }
    n88 = Equal?(x=w13, y="Exit") -> (x = y?=w11:bool)
  }
  "Initalized" <- w3
